vi "References fgv.vi"(7 "Set?":bool, 8 "error in (no error)":errorcluster, 11 "?":T1) -> (0 "error out":errorcluster, 3 "Cluster":T1)   [LabVIEW 2016]
uses:
  Controls/References.ctl
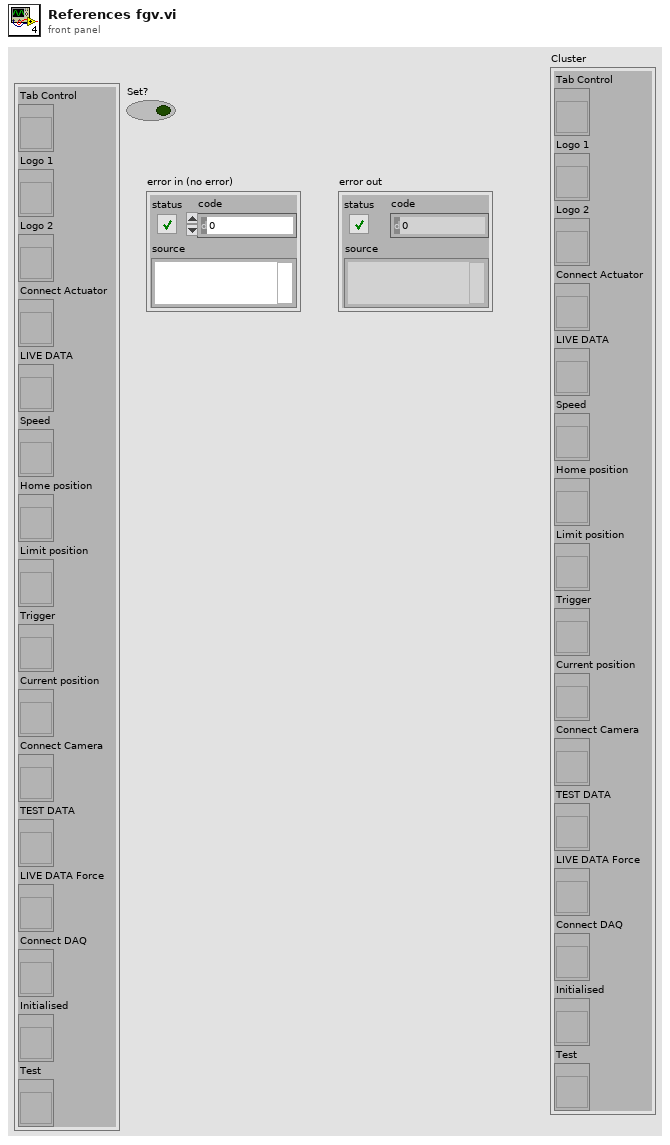
[diagram p1: front panel]
types:
  T1 = typedef "References.ctl" = cluster{"Tab Control":refnum<vi>, "Logo 1":refnum<vi>, "Logo 2":refnum<vi>, "Connect Actuator":refnum<vi>, "LIVE DATA":refnum<vi>, "Speed":refnum<vi>, "Home position":refnum<vi>, "Limit position":refnum<vi>, "Trigger":refnum<vi>, "Current position":refnum<vi>, "Connect Camera":refnum<vi>, "TEST DATA":refnum<vi>, "LIVE DATA Force":refnum<vi>, "Connect DAQ":refnum<vi>, "Initialised":refnum<vi>, "Test":refnum<vi>}
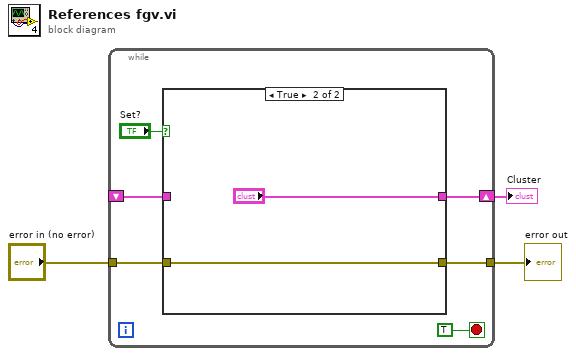
[diagram p0: block diagram]
diagram:
  n1 = while {
    shift-right: [w7] -> w3
    shift-left: _ -> [w6]
    tunnel: "error in (no error)" -> [w5]
    tunnel: [w4] -> w1
    stop <- TRUE stop-if-true
    n2 = case shown="True" "Set?" {
      tunnel: [w11 "?"] -> w7
      tunnel: w6 -> [w11 _]
      tunnel: w5 -> [w10 w12]
      tunnel: [w10 w12] -> w4
      frame False {
      }
      frame True {
      }
    }
  }
  "Cluster" <- w3
  "error out" <- w1
